vi "_builtins_distribute_selected.vi"(8 "error in (no error)":errorcluster, 9 "Distribute Type":T1, 10 "Panel":enum8{"FP", "BD"}(ring), 11 "VI Refnum in":refnum<vi>) -> (0 "error out":errorcluster, 3 "VI Refnum out":refnum<vi>)   [LabVIEW 2019, in "Script.lvlib"]
doc: "Distributes the selected front panel or block diagram objects including any display objects (i.e. labels, captions, inc/dec buttons, etc.)\n\nCreated by: Ryan Pacini"
uses:
  Script.lvlib
  _builtins_distribute.ctl
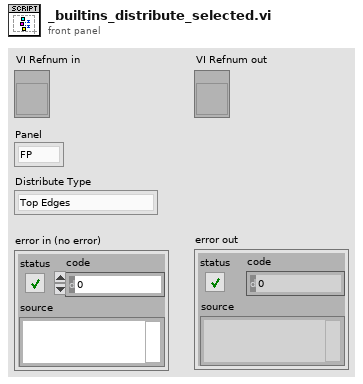
[diagram p1: front panel]
types:
  T1 = typedef "Script.lvlib/_builtins_distribute.ctl" = enum8{"Top Edges", "Vertical Centers", "Bottom Edges", "Vertical Gap", "Vertical Compress", "Left Edges", "Horizontal Centers", "Right Edges", "Horizontal Gap", "Horizontal Compress"}
  T2 = enum32{"Top Edges", "Vertical Centers", "Bottom Edges", "Vertical Gap", "Vertical Compress", "Left Edges", "Horizontal Centers", "Right Edges", "Horizontal Gap", "Horizontal Compress"}
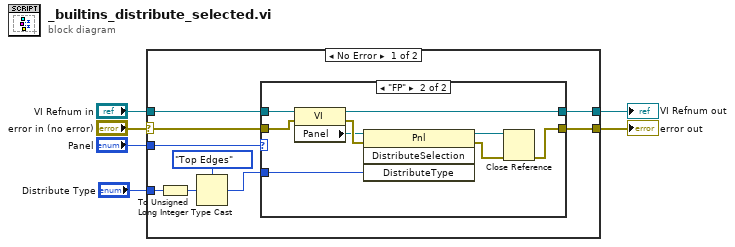
[diagram p0: block diagram]
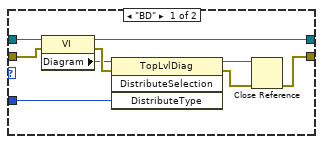
[diagram p2: hidden frame]
diagram:
  n1 = case shown="No Error" "error in (no error)" {
    selector: "error in (no error)" -> [w11 w34]
    tunnel: "Panel" -> [w15 _]
    tunnel: "VI Refnum in" -> [w14 w35]
    tunnel: [w13 w35] -> w4
    tunnel: [w12 w34] -> w3
    tunnel: "Distribute Type" -> [w10 _]
    frame No Error {
      n2 = To Unsigned Long Integer(number=w10) -> (unsigned 32bit integer=w7:u32)
      n3 = Type Cast(type=T2."Top Edges" ("DistributeType"), x=w7) -> (*(type *) &x=w9:T2)
      n4 = case shown="\"FP\"" w15 {
        tunnel: w11 -> [w23 w32]
        tunnel: w14 -> [w21 w30]
        tunnel: [w22 w31] -> w12
        tunnel: [w19 w28] -> w13
        tunnel: w9 -> [w16 w25]
        frame "BD" {
          n5 = property class="VI"(reference=w21, error in=w23) -> (reference out=w19:refnum<vi>, error out=w24:errorcluster, "Diagram"=w20:refnum<vi>)
          n6 = invoke class="TopLvlDiag" method="DistributeSelection"(reference=w20, error in=w24, "DistributeType"=w16) -> (reference out=w17:refnum<vi>, error out=w18:errorcluster)  [unwired: 1 in, 2 out]
          n7 = Close Reference(reference=w17, error in (no error)=w18) -> (error out=w22:errorcluster)
        }
        frame "FP" {
          n8 = property class="VI"(reference=w30, error in=w32) -> (reference out=w28:refnum<vi>, error out=w33:errorcluster, "Panel"=w29:refnum<vi>)
          n9 = invoke class="Pnl" method="DistributeSelection"(reference=w29, error in=w33, "DistributeType"=w25) -> (reference out=w26:refnum<vi>, error out=w27:errorcluster)  [unwired: 1 in, 2 out]
          n10 = Close Reference(reference=w26, error in (no error)=w27) -> (error out=w31:errorcluster)
        }
      }
    }
    frame Error {
    }
  }
  "VI Refnum out" <- w4
  "error out" <- w3
